vi "rsscope_FormatUSBPDPacketTypeString_ReadCallback.vi"(5 "Attribute":T1={"Identifier"="", "Descriptive Name"="", "Data Type"=enum."Integer 32", "Command"="", "Access"=enum."Read/Write", "Range Table"="", "Read Callback"="", "Write Callback"="", "Supported Models"="", "Instrument Options"="", "Index"=0, "OPC Wait"=FALSE, "No Status Check"=FALSE, "Cache Only"=FALSE}, 7 "Repeated Capability":string, 8 "error in (no error)":errorcluster, 11 "VISA resource name":refnum<visa-resource-name>) -> (0 "error out":errorcluster, 2 "Attribute Value String":string, 3 "VISA resource name out":refnum<visa-resource-name>)   [LabVIEW 2018]
doc: "This VI sets the attribute value.\n\nThis is a low-level VI that you can use to set the values of instrument-specific properties and inherent IVI properties. If the property represents an instrument state, this VI performs instrument I/O in the following cases:\n\n- State caching is disabled for the entire session or for the particular property.\n\n- State caching is enabled and the currently cached value is invalid or is different than the value you specify. \n\nThis instrument driver contains high-level VIs that set most of the instrument properties. It is best to use the high-level driver VIs as much as possible. They handle order dependencies and multithread locking for you. In addition, they perform status checking only after setting all of the properties. In contrast, when you set multiple properties using the SetAttribute VIs, the VIs check the instrument status after each call.\n\nAlso, when state caching is enabled, the high-level VIs that configure multiple properties perform instrument I/O only for the properties whose value you change. Thus, you can safely call the high-level VIs without the penalty of redundant instrument I/O."
uses:
  rsidr_core.llb/type_Attribute.ctl
  rsidr_core.llb/type_Attribute_Data_Type.ctl
  rsidr_core.llb/type_ReadWriteAccess.ctl
  rsidr_core.llb/rsscope_rsidr_core.lvlib
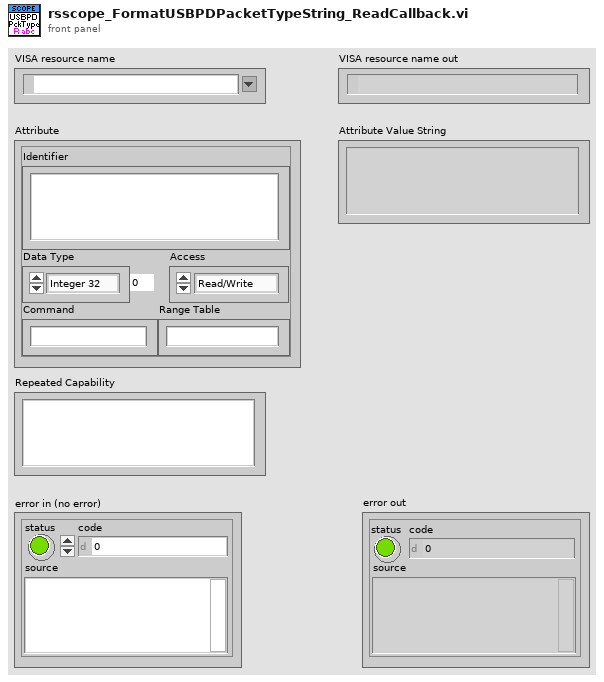
[diagram p1: front panel]
types:
  T1 = typedef "rsscope_rsidr_core.lvlib/type_Attribute.ctl" = cluster{"Identifier":string, "Descriptive Name":string, "Data Type":T2, "Command":string, "Access":T3, "Range Table":string, "Read Callback":string, "Write Callback":string, "Supported Models":string, "Instrument Options":string, "Index":i32, "OPC Wait":bool, "No Status Check":bool, "Cache Only":bool}
  T2 = typedef "rsscope_rsidr_core.lvlib/type_Attribute_Data_Type.ctl" = enum16{"Integer 32", "Double", "String", "Boolean", "None", "Integer 64", "RawString"}
  T3 = typedef "rsscope_rsidr_core.lvlib/type_ReadWriteAccess.ctl" = enum16{"Read Only", "Write Only", "Read/Write"}
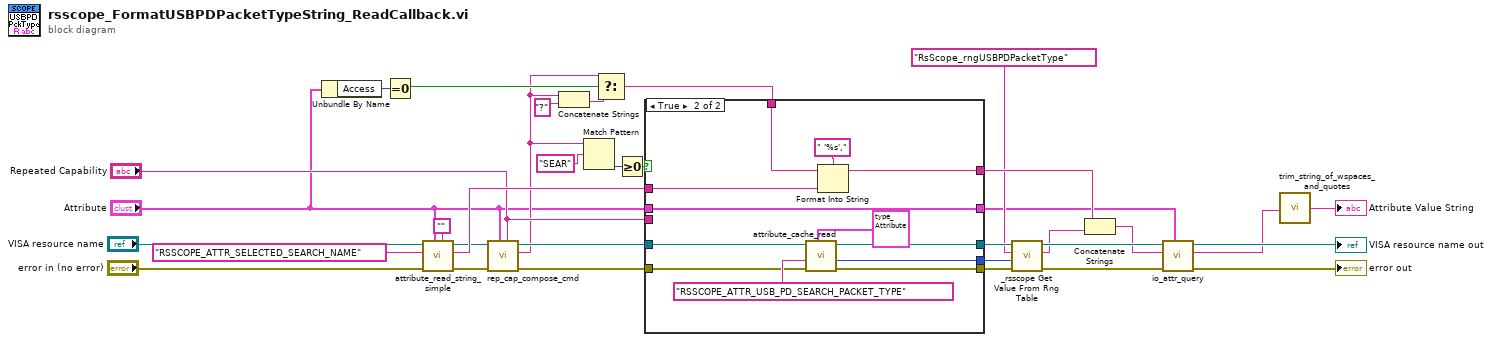
[diagram p0: block diagram]
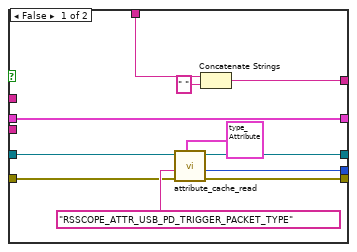
[diagram p2: hidden frame]
diagram:
  n1 = Unbundle By Name("Attribute") -> ("Access"=w23:T3)
  n2 = Equal To 0?(x=w23) -> (x = 0?=w22:bool)
  n3 = call "attribute_read_string_simple.vi"("Repeated Capability"="" ("Empty String Constant"), "Attribute"="Attribute", "error in"="error in (no error)", "Direct Attribute ID (\"\")"="RSSCOPE_ATTR_SELECTED_SEARCH_NAME" ("Direct Attribute ID (\"\")"), "VISA resource name"="VISA resource name") -> ("error out"=w30:errorcluster, "String out"=w29:string, "VISA resource name out"=w28:refnum<visa-resource-name>)  [unwired: 4 in]
  n4 = call "rep_cap_compose_cmd.vi"("Repeated Capability"="Repeated Capability", "Attribute"="Attribute", "error in"=w30, "VISA resource name"=w28) -> ("error out"=w19:errorcluster, "Command out"=w7:string, "VISA resource name out"=w20:refnum<visa-resource-name>)  [unwired: 5 in]
  n5 = Concatenate Strings(w7, "?" ("string")) -> (w25:string)
  n6 = Match Pattern(string=w7, regular expression="SEAR" ("true string")) -> (offset past match=w9:i32)  [unwired: 1 in, 3 out]
  n7 = Select(t=w7, s=w22, f=w25) -> (s? t:f=w21:string)
  n8 = Greater Or Equal To 0?(x=w9) -> (x >= 0?=w8:bool)
  n9 = case shown="True" w8 {
    tunnel: w29 -> [_ w56]
    tunnel: [w44 w55] -> w26
    tunnel: w21 -> [w45 w54]
    tunnel: w20 -> [w38 w48]
    tunnel: w19 -> [w39 w49]
    tunnel: [w36 w47] -> w17
    tunnel: [w37 w50] -> w16
    tunnel: [w35 w46] -> w15
    tunnel: "Repeated Capability" -> [_ _]
    tunnel: "Attribute" -> [w42 w53]
    tunnel: [w42 w53] -> w4
    frame False {
      n10 = call "attribute_cache_read.vi"("Attribute"=T1 {"Identifier"="", "Descriptive Name"="", "Data Type"=enum."Integer 32", "Command"="", "Access"=enum."Read/Write", "Range Table"="", "Read Callback"="", "Write Callback"="", "Supported Models"="", "Instrument Options"="", "Index"=0, "OPC Wait"=FALSE, "No Status Check"=FALSE, "Cache Only"=FALSE}, "error in"=w39, "Direct Attribute ID (Attribute cluster)"="RSSCOPE_ATTR_USB_PD_TRIGGER_PACKET_TYPE" ("Direct Attribute ID (\"\")"), "VISA resource name"=w38) -> ("error out"=w37:errorcluster, "Int32 out"=w35:i32, "VISA resource name out"=w36:refnum<visa-resource-name>)  [unwired: 5 out]
      n11 = Concatenate Strings(w45, " " ("string")) -> (w44:string)
    }
    frame True {
      n12 = call "attribute_cache_read.vi"("Attribute"=T1 {"Identifier"="", "Descriptive Name"="", "Data Type"=enum."Integer 32", "Command"="", "Access"=enum."Read/Write", "Range Table"="", "Read Callback"="", "Write Callback"="", "Supported Models"="", "Instrument Options"="", "Index"=0, "OPC Wait"=FALSE, "No Status Check"=FALSE, "Cache Only"=FALSE}, "error in"=w49, "Direct Attribute ID (Attribute cluster)"="RSSCOPE_ATTR_USB_PD_SEARCH_PACKET_TYPE" ("Direct Attribute ID (\"\")"), "VISA resource name"=w48) -> ("error out"=w50:errorcluster, "Int32 out"=w46:i32, "VISA resource name out"=w47:refnum<visa-resource-name>)  [unwired: 5 out]
      n13 = Format Into String(format string=" '%s',", initial string=w54, w56) -> (resulting string=w55:string)  [unwired: 1 in, 1 out]
    }
  }
  n14 = call "_rsscope Get Value From Rng Table.vi"("error in (no error)"=w16, "Value"=w15, "Range Table Name"="RsScope_rngUSBPDPacketType", "VISA resource name"=w17) -> ("error out"=w14:errorcluster, "Output Enum value"=w10:string, "VISA resource name out"=w13:refnum<visa-resource-name>)  [unwired: 5 in]
  n15 = Concatenate Strings(w26, w10) -> (w11:string)
  n16 = call "io_attr_query.vi"("Attribute"=w4, "error in"=w14, "write buffer"=w11, "VISA resource name"=w13) -> ("error out"=→"error out":errorcluster, "read buffer"=w1:string, "VISA resource name out"=→"VISA resource name out":refnum<visa-resource-name>)  [unwired: 5 in]
  n17 = call "trim_string_of_wspaces_and_quotes.vi"("String in"=w1) -> ("String out"=→"Attribute Value String":string)  [unwired: 4 in]
